vi "Configure Report Generator.vi"(8 "error in (no error)":errorcluster, 11 "Report Generator In":refnum<class "Report Generator.lvclass">) -> (0 "error out":errorcluster, 3 "Report Generator Out":refnum<class "Report Generator.lvclass">)   [LabVIEW 2020, in "Reports.lvlib" / "Report Generator.lvclass"]
uses:
  Report Generator.lvclass
  C:/git/astemes-lunit/source/User Interface/Process/Process.lvclass
  User Interface/Process/Process.lvclass/Process.ctl
  User Interface/Process/Protected/Enqueue Message.vi
  <vilib>/Utility/sysdir.llb/Get System Directory.vi
  <vilib>/Utility/libraryn.llb/Create Directory Recursive.vi
  Report Generator.lvclass/Report Generator.ctl
  User Interface/Configuration Manager/Configuration Manager.lvclass
  User Interface/Support/Paths.lvlib
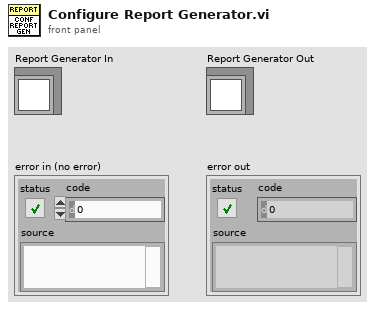
[diagram p1: front panel]
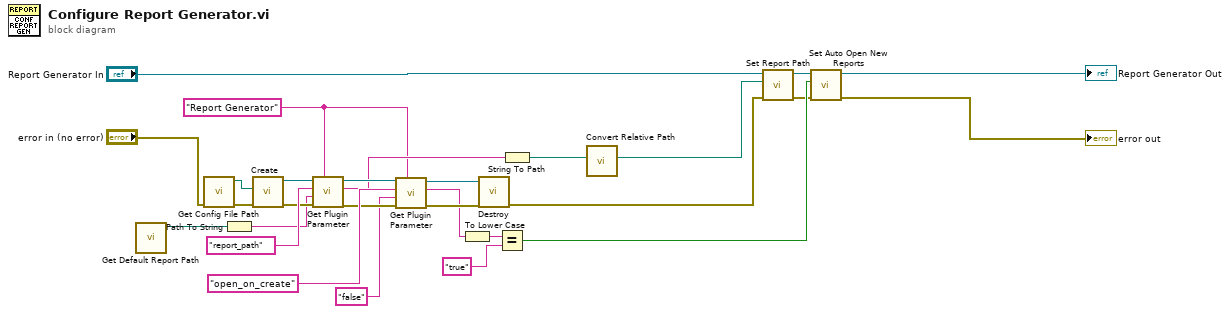
[diagram p0: block diagram]
diagram:
  w3 = "Report Generator"
  n1 = call "Get Default Report Path.vi"() -> ("Default Report Path"=w5:path)  [unwired: 10 in, 1 out]
  n2 = call "Get Config File Path.vi"("error in (no error)"="error in (no error)") -> ("error out"=w11:errorcluster, "Config Directory"=w15:path)  [unwired: 9 in]
  n3 = Path To String(path=w5) -> (string=w4:string)
  n4 = call "Create.vi"("error in (no error)"=w11, "configuration file path"=w15) -> ("error out"=w13:errorcluster, "Configuration Manager out"=w12:refnum<class "Configuration Manager.lvclass">)  [unwired: 8 in]
  n5 = call "Get Plugin Parameter.vi"("Plugin"=w3, "error in (no error)"=w13, "Default Value"=w4, "Name"="report_path", "Configuration Manager in"=w12) -> ("error out"=w14:errorcluster, "Value"=w16:string, "Configuration Manager out"=w20:refnum<class "Configuration Manager.lvclass">)  [unwired: 4 in]
  n6 = call "Get Plugin Parameter.vi"("Plugin"=w3, "error in (no error)"=w14, "Default Value"="false", "Name"="open_on_create", "Configuration Manager in"=w20) -> ("error out"=w19:errorcluster, "Value"=w7:string, "Configuration Manager out"=w21:refnum<class "Configuration Manager.lvclass">)  [unwired: 4 in]
  n7 = To Lower Case(string=w7) -> (all lower case string=w24:string)
  n8 = call "Destroy.vi"("error in (no error)"=w19, "Configuration Manager In"=w21) -> ("error out"=w8:errorcluster)  [unwired: 9 in]
  n9 = Equal?(x=w24, y="true") -> (x = y?=w26:bool)
  n10 = String To Path(string=w16) -> (path=w2:path)
  n11 = call "Convert Relative Path.vi"("File Path in"=w2) -> ("Modified Path"=w1:path)  [unwired: 10 in]
  n12 = call "Set Report Path.vi"("error in (no error)"=w8, "Report Directory"=w1, "Report Generator In"="Report Generator In") -> ("error out"=w10:errorcluster, "Report Generator Out"=w18:refnum<class "Report Generator.lvclass">)  [unwired: 7 in]
  n13 = call "Set Auto Open New Reports.vi"("error in (no error)"=w10, "Open New Reports?"=w26, "Report Generator In"=w18) -> ("error out"=→"error out":errorcluster, "Report Generator Out"=→"Report Generator Out":refnum<class "Report Generator.lvclass">)  [unwired: 7 in]
